vi "Simple-TCP.vi"() -> ()   [LabVIEW 2020]
doc: "创建一个命名服务并在第一个可用端口侦听。当客户端连接该服务时，将发送一个响应字符串至客户端。"
panel:
  in  "停止":bool
  out "波形图表 3":i32(graph)
  # "概述：演示使用TCP函数初始化可向客户端VI发送数据的命名TCP服务。\n操作步骤:\n1.运行VI。\n2.打开TCP Named Service - Client.vi并按照前面板上的说明操作。\n3.单击停止 停止VI运行。"
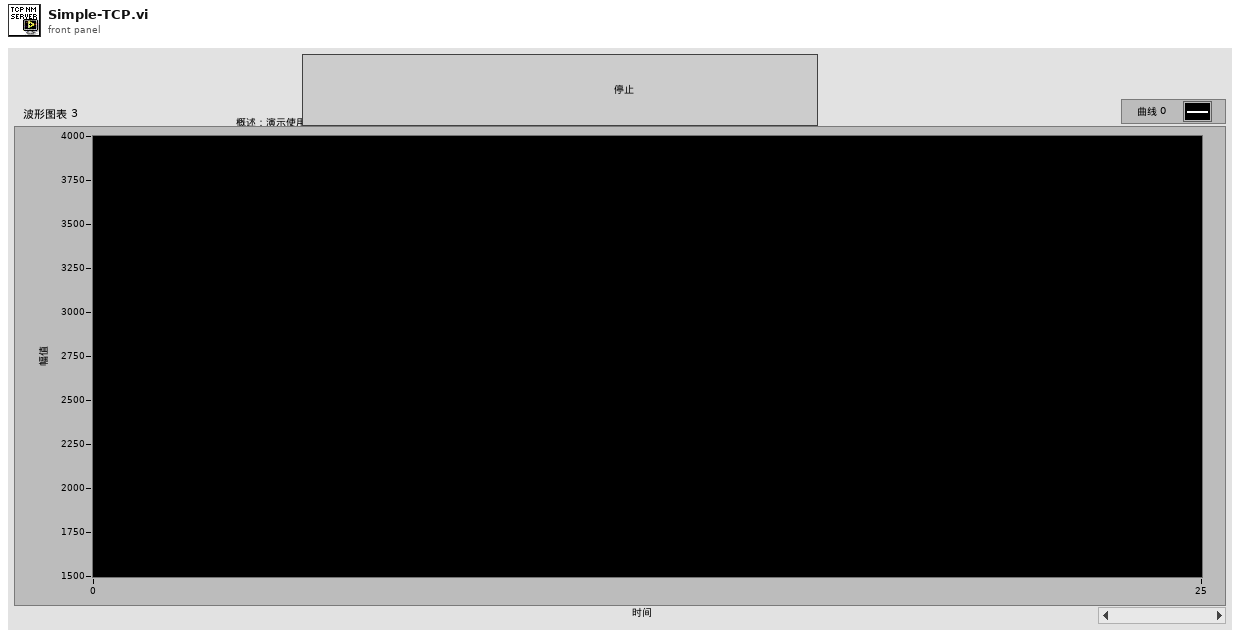
[diagram p1: front panel]
types:
  T1 = enum16{"open", "open or create", "create or replace", "create", "open (read-only)"}
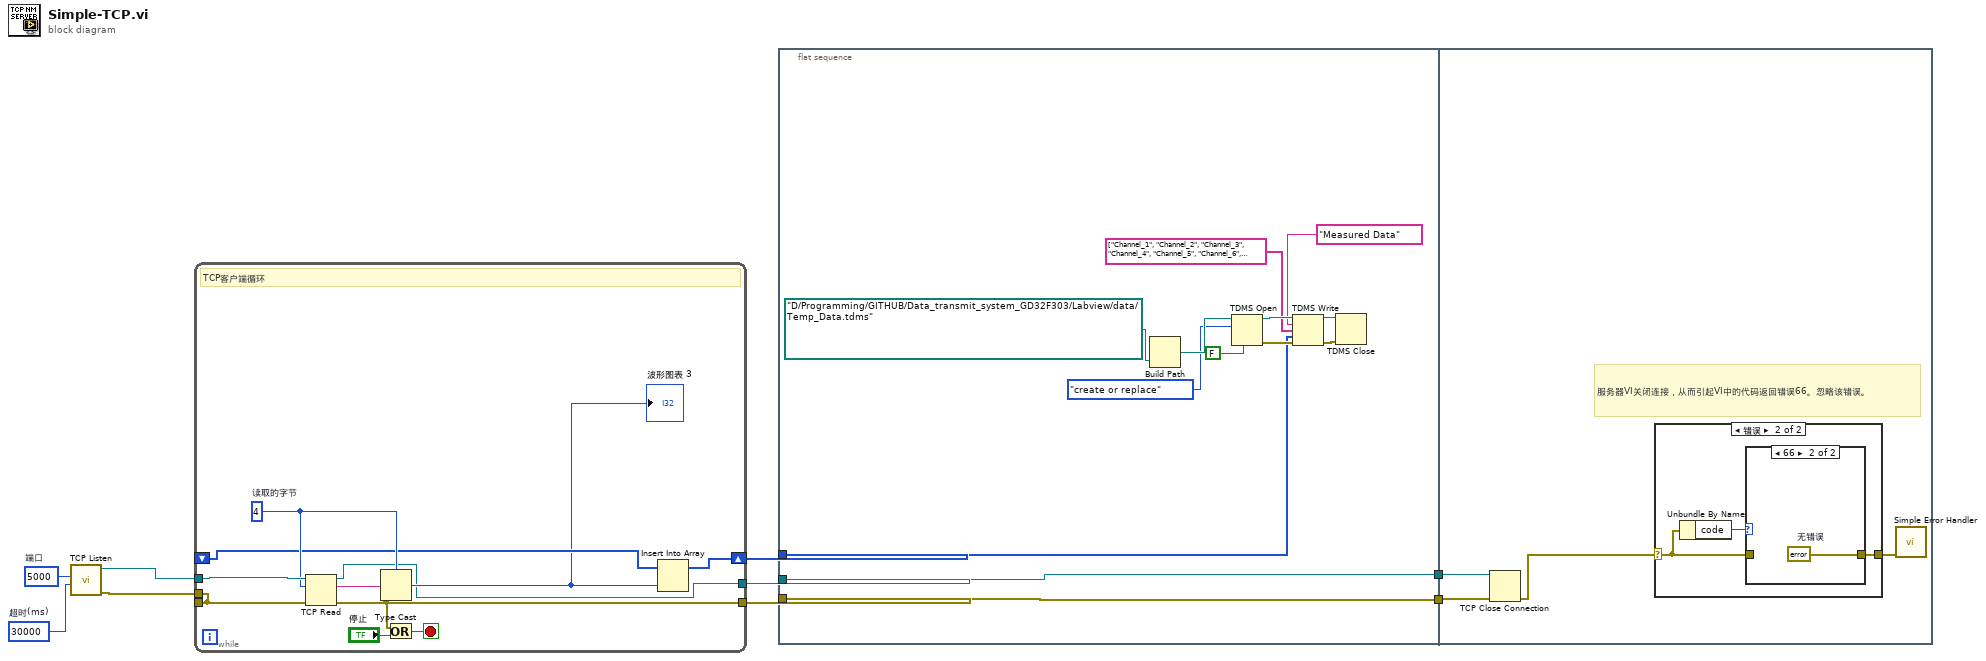
[diagram p0: block diagram]
diagram:
  w8 = u16 5000  # 端口
  w9 = 30000  # 超时(ms)
  n1 = call <vilib>:"TCP Listen.vi"("timeout ms (wait forever: -1)"=w9, "port"=w8) -> ("error out"=w6:errorcluster, "connection ID"=w7:refnum<k5>)  [unwired: 5 in, 3 out]
  n2 = while {
    tunnel: [w16] -> _
    tunnel: w7 -> [w20]
    tunnel: [w17] -> w3
    tunnel: w6 -> [w16]
    shift-right: [w13] -> w5
    shift-left: _ -> [w12]
    tunnel: [w10] -> w2
    stop <- w18 stop-if-true
    w14 = 4  # 读取的字节
    # "TCP客户端循环"
    n3 = TCP Read(connection ID=w20, bytes to read=w14, error in (no error)=w16) -> (connection ID out=w10:refnum<k5>, data out=w15:string, error out=w17:errorcluster)  [unwired: 2 in]
    n4 = Type Cast(type=w14, x=w15) -> (*(type *) &x=w11:i32)
    "波形图表 3" <- w11
    n5 = Or(x=w17, y="停止") -> (x .or. y?=w18:bool)
    n6 = Insert Into Array(array=w12, new element=w11) -> (w13:i32[])  [unwired: 1 in]
  }
  n7 = flat-sequence {
    tunnel: w5 -> [w23]
    tunnel: [w22] -> w4
    tunnel: w3 -> [w22]
    tunnel: w2 -> [w21]
    tunnel: [w21] -> w1
    tunnel: w4 -> [w37]
    tunnel: w1 -> [w36]
    frame #0 {
      n8 = Build Path(name or relative path=path "D:/Programming/GITHUB/Data_transmit_system_GD32F303/Labview/data/Temp_Data.tdms" ("file path")) -> (appended path=w29:path)  [unwired: 1 in]
      n9 = TDMS Open(6:FALSE ("disable buffering (T)"), 10:T1."create or replace" ("operation"), 11:w29) -> (0:w33:errorcluster, 3:w30:refnum<k34>)  [unwired: 4 in]
      n10 = TDMS Write(0:w30, 5:"Measured Data" ("group name"), 7:string[] ["Channel_1", "Channel_2", "Channel_3", "Channel_4", "Channel_5", "Channel_6", "Channel_7", "Channel_8", "Channel_9", "Channel_10", "Channel_11", "Channel_12", "Channel_13", "Channel_14", "Channel_15", "Channel_16"] ("channel names"), 9:w23, 11:w33) -> (4:w31:refnum<k34>, 15:w32:errorcluster)  [unwired: 1 in, 2 out]
      n11 = TDMS Close(8:w32, 11:w31) -> ()  [unwired: 2 out]
    }
    frame #1 {
      # "服务器VI关闭连接，从而引起VI中的代码返回错误66。忽略该错误。"
      n12 = TCP Close Connection(connection ID=w36, error in (no error)=w37) -> (error out=w34:errorcluster)  [unwired: 1 in, 1 out]
      n13 = case shown="错误" w34 {
        selector: w34 -> [w38 w40]
        tunnel: [w38 w39] -> w35
        frame No Error {
        }
        frame Error {
          n14 = Unbundle By Name(w40) -> ("code"=w41:i32)
          n15 = case shown="66" w41 {
            tunnel: w40 -> [w42 _]
            tunnel: [w42 w43] -> w39
            frame Default {
            }
            frame 66 {
              w43 = errorcluster {"status"=FALSE, "code"=0, "source"=""}  # 无错误
            }
          }
        }
      }
      n16 = call <vilib>:"Simple Error Handler.vi"("error in (no error)"=w35) -> ()  [unwired: 4 in, 5 out]
    }
  }
